vi "GA_Select Parent.vi"(6 "Parameters":T1={"Population size"=100, "Generations no."=500, "Significant digits"=4, "Crossover probabality"=0.85, "Mutation mode"=enum."one-point, fixed rate", "Use Gray code?"=FALSE, "Mutation rate"=0.05, "Min mutation rate"=0.0005, "Max mutation rate"=0.25, "Reproduction plan"=enum."Steady-state-replace-worst", "Elitism"=FALSE, "Fmax"=1} {"Max mutation rate" min=0.0 max=1.0; "Min mutation rate" min=0.0 max=1.0; "Mutation rate" min=0.0 max=1.0; "Crossover probabality" min=0.0 max=1.0; "Significant digits" min=1; "Generations no." min=1; "Population size" min=1}, 11 "Ranks":i32[](array[numeric])) -> (3 "Parent index":i32)   [LabVIEW 2016, in "Optimal Frequency Bands Search.lvlib" / "GeneticAlgorithm.lvlib"]
doc: "Выбрать родительскую особь из популяции"
uses:
  GeneticAlgorithm.lvlib
  GA_tParameters.ctl
panel:
  # "This VI is a part of BCI Design library, http://www.ru-bci.org \nCopyright © 2020, Sotnikov Peter, All rights reserved. License: GNU GPLv3"
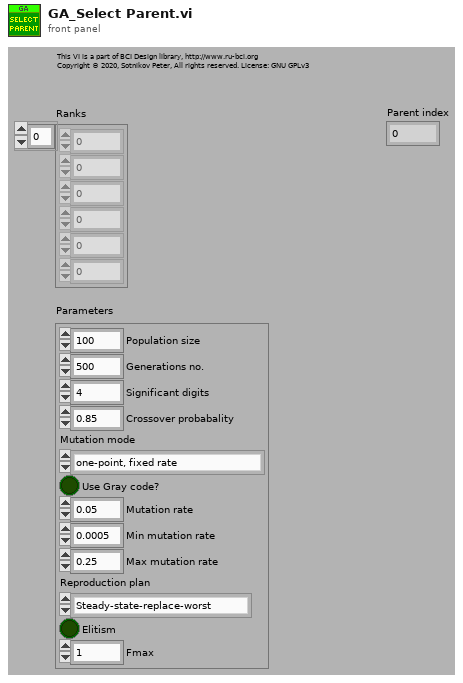
[diagram p1: front panel]
types:
  T1 = typedef "Optimal Frequency Bands Search.lvlib/GeneticAlgorithm.lvlib/GA_tParameters.ctl" = cluster{"Population size":i32, "Generations no.":i32, "Significant digits":i32, "Crossover probabality":dbl, "Mutation mode":enum16{"one-point, fixed rate", "one-point, fitness-adjustable rate", "one-point, distance-adjustable rate"}, "Use Gray code?":bool, "Mutation rate":dbl, "Min mutation rate":dbl, "Max mutation rate":dbl, "Reproduction plan":enum16{"Full generational replacement", "Steady-state-replace-random", "Steady-state-replace-worst"}, "Elitism":bool, "Fmax":i32}
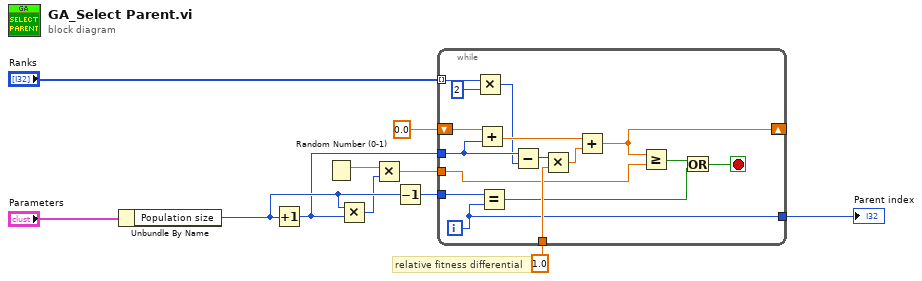
[diagram p0: block diagram]
diagram:
  # "relative fitness differential"
  n1 = Unbundle By Name("Parameters") -> ("Population size"=w9:i32)
  n2 = Increment(x=w9) -> (x+1=w3:i32)
  n3 = Random Number (0-1)() -> (number: 0 to 1=w8:dbl)
  n4 = Multiply(x=w9, y=w3) -> (x*y=w7:i32)
  n5 = Multiply(x=w8, y=w7) -> (x*y=w5:dbl)
  n6 = Decrement(x=w9) -> (x-1=w2:i32)
  n7 = while {
    tunnel: "Ranks" -> [w13] mode=indexing
    tunnel: w2 -> [w27]
    tunnel: w5 -> [w18]
    shift-right: [w19] -> _
    shift-left: 0.0 -> [w26]
    tunnel: w3 -> [w24]
    tunnel: 1.0 ("Relative fitness differential") -> [w22]
    tunnel: [w12] -> w10
    i -> [w12]
    stop <- w15 stop-if-true
    n8 = Multiply(x=w13, y=2) -> (x*y=w14:i32)
    n9 = Add(x=w26, y=w24) -> (x+y=w21:dbl)
    n10 = Equal?(x=w27, y=w12) -> (x = y?=w16:bool)
    n11 = Subtract(x=w24, y=w14) -> (x-y=w23:i32)
    n12 = Multiply(x=w23, y=w22) -> (x*y=w20:dbl)
    n13 = Add(x=w21, y=w20) -> (x+y=w19:dbl)
    n14 = Greater Or Equal?(x=w19, y=w18) -> (x >= y?=w17:bool)
    n15 = Or(x=w17, y=w16) -> (x .or. y?=w15:bool)
  }
  "Parent index" <- w10
